vi "Pause milliGAT.vi"(8 "error in (no error)":errorcluster, 10 "Letter Enum":refnum<vi>, 11 "VICI Settings in":T1) -> (0 "error out":errorcluster, 3 "VICI Settings out":T1)   [LabVIEW 2018, in "VICI M6 M50 Party Mode.lvlib"]
uses:
  VICI M6 M50 Party Mode.lvlib
  \\smbgbl.drmvfs102.pfizer.com\FAST_Team/Software/LabVIEW/Third Party Drivers/Third Party Drivers/VICI/Global FIA milliGAT.lvlib
  Settings Cluster.ctl
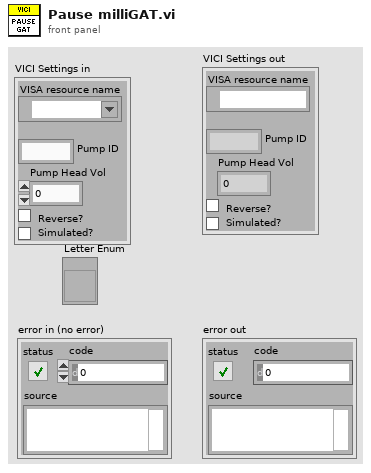
[diagram p1: front panel]
types:
  T1 = typedef "VICI M6 M50 Party Mode.lvlib/Settings Cluster.ctl" = cluster{"VISA resource name":refnum<visa-resource-name>, "Pump ID":string, "Pump Head Vol":dbl, "Reverse?":bool, "Simulated?":bool}
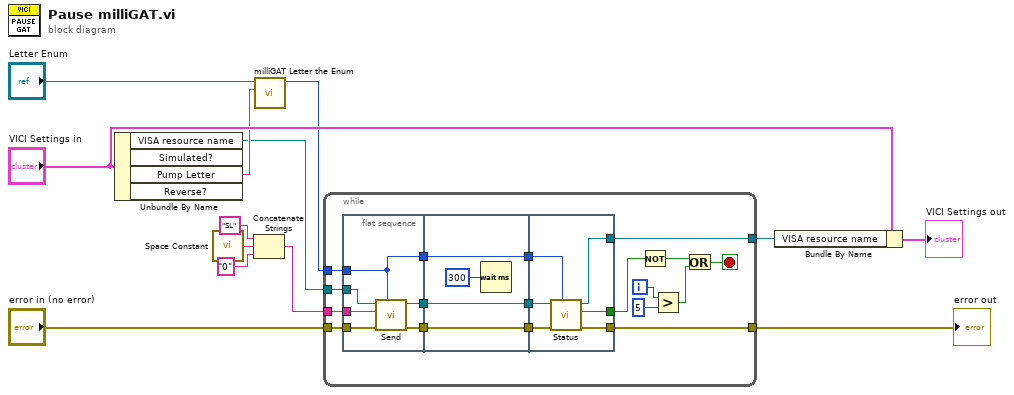
[diagram p0: block diagram]
diagram:
  n1 = Unbundle By Name("VICI Settings in") -> ("VISA resource name"=w6:refnum<visa-resource-name>, "Pump Letter"=w8:string)  [unwired: 2 out]
  n2 = call <vilib>:"Space Constant.vi"() -> ("String"=w2:string)
  n3 = Concatenate Strings("SL", w2, "0" ("string")) -> (w3:string)
  n4 = call "milliGAT Letter the Enum.vi"("Pump Letter"=w8, "Enum in"="Letter Enum") -> ("Numeric"=w9:i32)  [unwired: 9 in]
  n5 = while {
    tunnel: w3 -> [w31]
    tunnel: "error in (no error)" -> [w30]
    tunnel: w6 -> [w29]
    tunnel: w9 -> [w28]
    tunnel: [w17] -> w11
    tunnel: [w16] -> w12
    i -> [w21]
    stop <- w18 stop-if-true
    n6 = flat-sequence {
      tunnel: w31 -> [w37]
      tunnel: w30 -> [w36]
      tunnel: w29 -> [w35]
      tunnel: w28 -> [w32]
      tunnel: [w34] -> w26
      tunnel: [w33] -> w24
      tunnel: [w32] -> w15
      tunnel: [w40] -> w27
      tunnel: w26 -> [w40]
      tunnel: [w39] -> w25
      tunnel: w24 -> [w39]
      tunnel: w15 -> [w38]
      tunnel: [w38] -> w14
      tunnel: w27 -> [w47]
      tunnel: w25 -> [w46]
      tunnel: [w45] -> w23
      tunnel: [w44] -> w17
      tunnel: [w43] -> w16
      tunnel: w14 -> [w42]
      frame #0 {
        n7 = call "Send.vi"("Pump ID (0:A)"=w32, "error in (no error)"=w36, "Command"=w37, "VISA resource in"=w35) -> ("error out"=w34:errorcluster, "VISA resource out"=w33:refnum<visa-resource-name>)  [unwired: 5 in, 1 out]
      }
      frame #1 {
        n8 = Wait (ms)(milliseconds to wait=u32 300) -> ()  [unwired: 1 out]
      }
      frame #2 {
        n9 = call "Status.vi"("Pump ID (0:A)"=w42, "error in (no error)"=w47, "VISA resource in"=w46) -> ("error out"=w43:errorcluster, "moving"=w45:bool, "VISA resource out"=w44:refnum<visa-resource-name>)  [unwired: 6 in]
      }
    }
    n10 = Not(x=w23) -> (.not. x?=w22:bool)
    n11 = Greater?(x=w21, y=5) -> (0:w19:bool)
    n12 = Or(x=w22, y=w19) -> (x .or. y?=w18:bool)
  }
  "error out" <- w12
  n13 = Bundle By Name(cluster="VICI Settings in", "VISA resource name"=w11) -> (→"VICI Settings out":T1)
